vi "Autonomous Independent.vi"   [LabVIEW 2015]
doc: "This VI is called when autonomous begins, and will automatically be terminated when autonomous ends. You can carry out timed or sensor driven robot movement independently without needing to return to the caller."
uses:
  <vilib>/Rock Robotics/WPI/SafetyOutput/WPI_SafetyOutputConfigMenu.ctl
  <vilib>/Rock Robotics/Network Tables/NT Read String.vi
  <vilib>/Rock Robotics/WPI/Utilities/WPI_GetSetVariantRefNum.vi
  <vilib>/addons/control/pid/pid.llb/PID (DBL).vi
  Z navX/navX Library v2/navX Library v2.lvlib
  <vilib>/addons/control/pid/NI_PID_pid.lvlib
panel:
  # "Be sure to right-click and choose Data Operations>>Make Current Value default if you want to save the array values with the VI"
types:
  T1 = cluster{"proportional gain (Kc)":dbl, "integral time (Ti, min)":dbl, "derivative time (Td, min)":dbl}
  T2 = typedef "WPI_SafetyOutputConfigMenu.ctl" = enum16{"Enable", "Disable"}
  T3 = typedef "navX Library v2.lvlib/Z900_navX_DeviceTypeDef.ctl" = cluster{"Interface":cluster{"Protocol":T4, "Update Rate (4Hz-60Hz)":u8, "navX Open TypeDef":variant}, "Notify Packet":refnum<notifier>, "Loop VI Refnum":refnum<vi>, "Ready to Close Occurrence Refnum":refnum<k4>}
  T4 = typedef "navX Library v2.lvlib/Z900_navX_ProtocolTypeDef.ctl" = enum16{"SERIAL", "I2C", "SPI"}
  T5 = cluster{"LinearAcceleration X":dbl, "LinearAcceleration Y":dbl, "LinearAcceleration Z":dbl}
  T6 = cluster{"Velocity X":dbl, "Velocity Y":dbl, "Velocity Z":dbl, "Displacement X":dbl, "Displacement Y":dbl, "Displacement Z":dbl}
  T7 = cluster{"Yaw":dbl, "Roll":dbl, "Pitch":dbl, "Heading":dbl, "Fused Heading":dbl}
  T8 = typedef "WPI_RobotDriveDevRef.ctl" = cluster{"DevStatus":errorcluster, "Motors[]":T9[], "Square Inputs":bool, "Max Output":dbl}
  T9 = typedef "WPI_MotorControlDeviceRef.ctl" = cluster{"DeviceStatus":errorcluster, "Type":T10, "PWM":cluster{"PWM Channel":T11, "DeadBand":T12}, "CAN":cluster{"Device Number":u8, "Control Mode":T13, "Semaphore":T14, "Max Vout":dbl, "TalonSRX Control Mode":T15}, "Invert":bool}
  T10 = typedef "WPI_MotorControlType.ctl" = enum16{"PWM", "CAN", "CANTalonSRX"}
  T11 = typedef "FPGA_DIOPWMChannel.ctl" = enum8{"PWM 0", "PWM 1", "PWM 2", "PWM 3", "PWM 4", "PWM 5", "PWM 6", "PWM 7", "PWM 8", "PWM 9", "PWM MXP 0", "PWM MXP 1", "PWM MXP 2", "PWM MXP 3", "PWM MXP 4", "PWM MXP 5", "PWM MXP 6", "PWM MXP 7", "PWM MXP 8", "PWM MXP 9", "Invalid"}
  T12 = typedef "WPI_PWMDeadband.ctl" = cluster{"Name":string, "maxPositivePwm":i32, "minPositivePwm":i32, "centerPwm":i32, "maxNegativePwm":i32, "minNegativePwm":i32, "angularRange":u16}
  T13 = typedef "WPI_CANJaguar_ControlMode.ctl" = enum8{"Percent VBus", "Current", "Speed", "Position", "Voltage"}
  T14 = typedef "Semaphore RefNum" = refnum<k1>
  T15 = typedef "WPI_CANTalonSRX_APIControlMode.ctl" = enum8{"Percent VBus", "Speed", "Position", "Slave", "Unchanged / Invalid", "Voltage Compensation", "Current", "Motion Profile"}
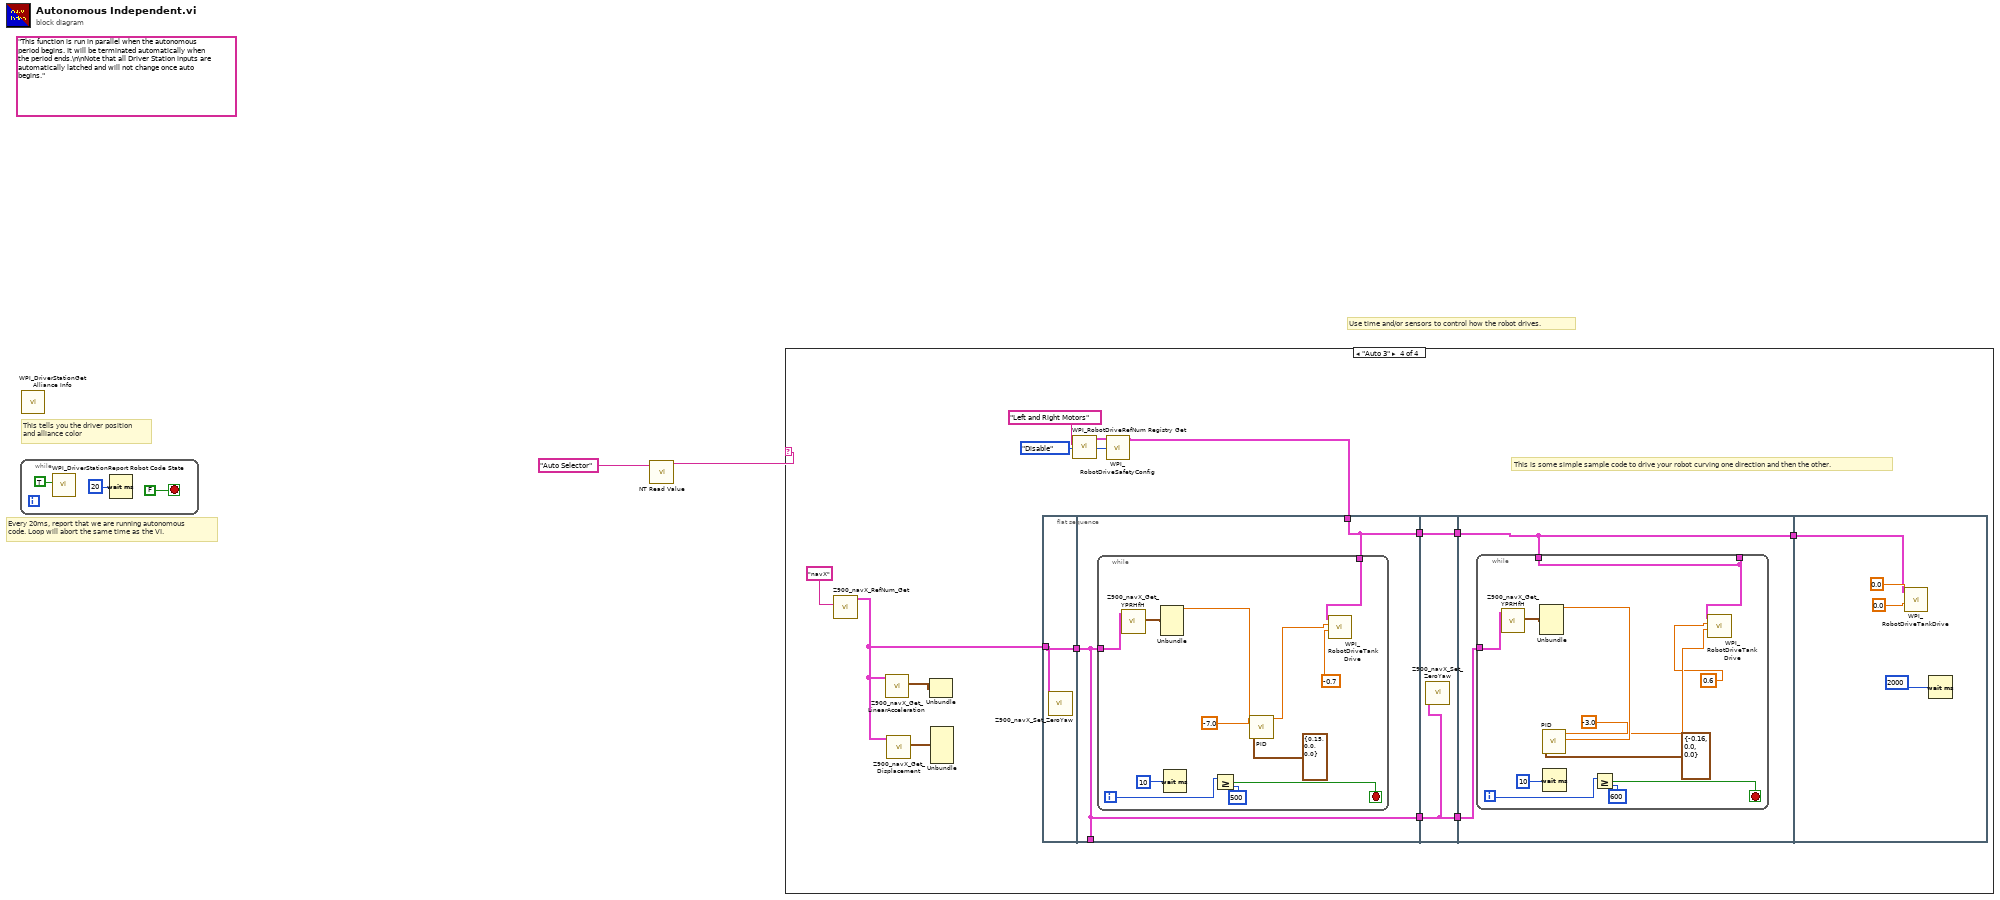
[diagram p0: block diagram]
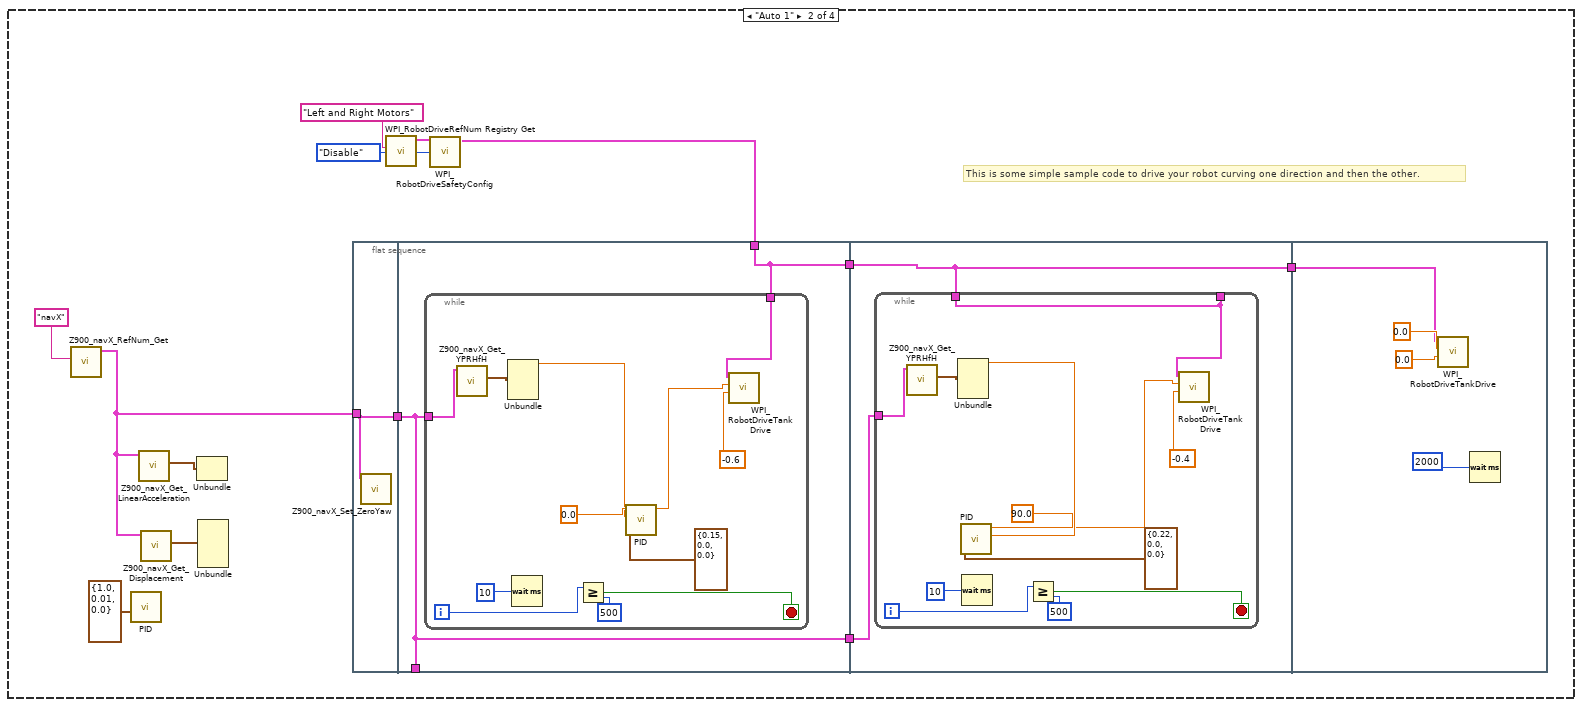
[diagram p3: hidden frame]
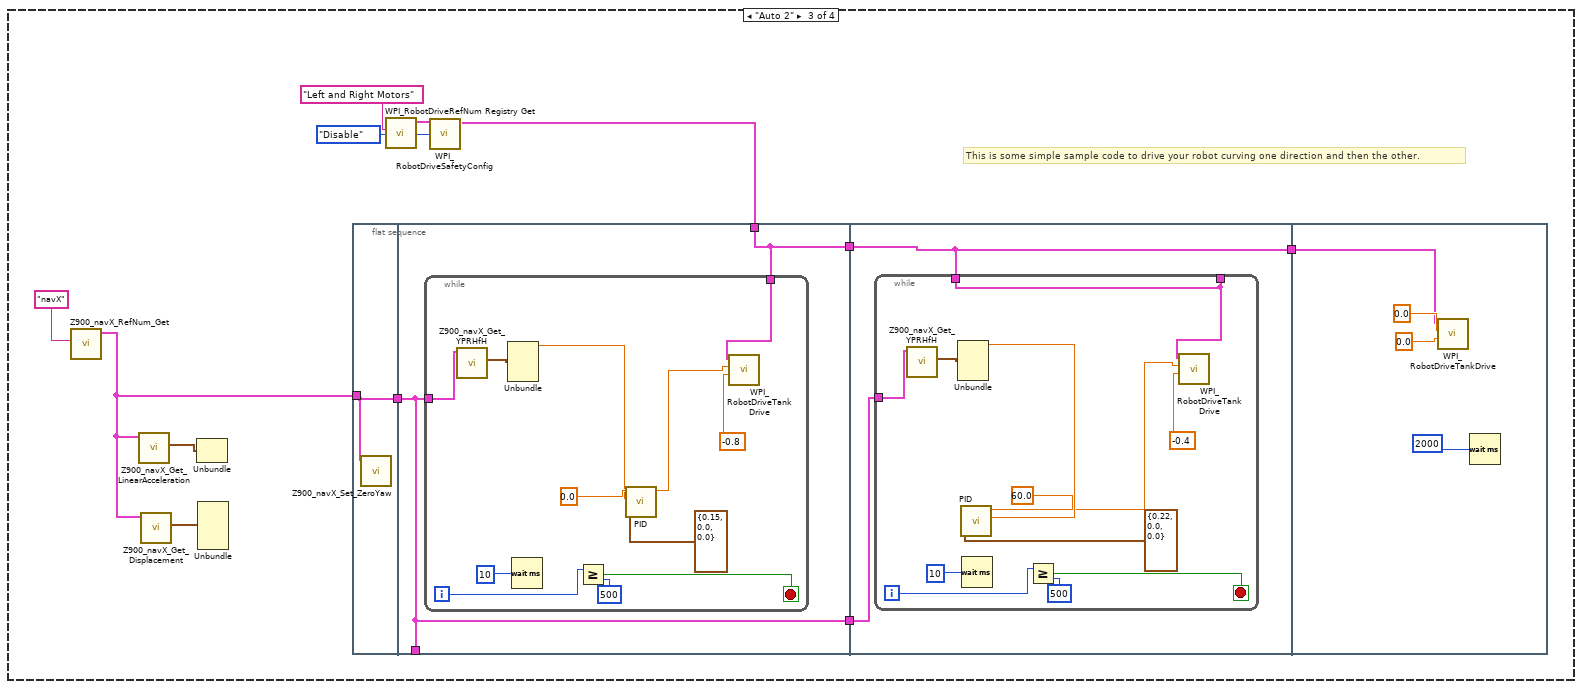
[diagram p4: hidden frame]
diagram:
  (unwired) "This function is run in parallel when the autonomous period begins. It will be terminated automatically when the period ends.\n\nNote that all Driver Station inputs are automatically latched and will not change once auto begins."
  # "Use time and/or sensors to control how the robot drives."
  # "Every 20ms, report that we are running autonomous\ncode. Loop will abort the same time as the VI."
  # "This tells you the driver position\nand alliance color"
  n1 = while {
    stop <- FALSE stop-if-true
    n2 = call <vilib>:"WPI_DriverStationReport Robot Code State.vi"("Autonomous"=TRUE) -> ()  [unwired: 10 in, 1 out]
    n3 = Wait (ms)(milliseconds to wait=u32 20) -> ()  [unwired: 1 out]
  }
  n4 = call <vilib>:"WPI_DriverStationGet Alliance Info.vi"() -> ()  [unwired: 12 out]
  n5 = call-poly <vilib>:"NT Read Value.vi"("Name"="Auto Selector") -> ("String"=w1:string)  [unwired: 9 in, 1 out]
  n6 = case shown="\"Auto 3\"" w1 {
    frame Default {
      # "You can put your main auto here, or you can right-click on the case and make any\nother frame be the default case."
      # "This is the frame that will execute if no selection is made, or if it is not recognized"
    }
    frame "Auto 1" {
      # "This is some simple sample code to drive your robot curving one direction and then the other."
      n7 = call "Z900_navX_RefNum_Get.vi"("refnum name"="navX") -> ("navX Device"=w9:T3)  [unwired: 9 in, 1 out]
      n8 = call-poly <vilib>:"PID.vi"("PID gains"=T1 {"proportional gain (Kc)"=1.0, "integral time (Ti, min)"=0.01, "derivative time (Td, min)"=0.0}) -> ()  [unwired: 9 in, 2 out]
      n9 = call "Z900_navX_Get_LinearAcceleration.vi"("navX Device"=w9) -> ("Linear Acceleration"=w11:T5)  [unwired: 7 in, 3 out]
      n10 = call "Z900_navX_Get_Displacement.vi"("navX Device"=w9) -> ("Displacement"=w10:T6)  [unwired: 7 in, 3 out]
      n11 = Unbundle(w11) -> ()  [unwired: 3 out]
      n12 = Unbundle(w10) -> ()  [unwired: 6 out]
      n13 = flat-sequence {
        tunnel: w9 -> [w19]
        tunnel: [w19] -> w7
        tunnel: w14 -> [w21]
        tunnel: [w21] -> w18
        tunnel: w7 -> [w20]
        tunnel: [w20] -> _
        tunnel: [w20] -> w6
        tunnel: w18 -> [w35]
        tunnel: [w35] -> w13
        tunnel: w6 -> [w34]
        tunnel: w13 -> [w48]
        frame #0 {
          n14 = call "Z900_navX_Set_ZeroYaw.vi"("navX Device"=w19) -> ()  [unwired: 9 in, 2 out]
        }
        frame #1 {
          n15 = while {
            tunnel: w21 -> [w30]
            tunnel: w20 -> [w25]
            i -> [w29]
            stop <- w27 stop-if-true
            n16 = call "Z900_navX_Get_YPRHfH.vi"("navX Device"=w25) -> ("YRPHfH"=w26:T7)  [unwired: 7 in, 3 out]
            n17 = Unbundle(w26) -> ("Yaw"=w22:dbl)  [unwired: 4 out]
            n18 = Wait (ms)(milliseconds to wait=10) -> ()  [unwired: 1 out]
            n19 = Greater Or Equal?(x=w29, y=500) -> (x >= y?=w27:bool)
            n20 = call-poly <vilib>:"PID.vi"("PID gains"=T1 {"proportional gain (Kc)"=0.15, "integral time (Ti, min)"=0.0, "derivative time (Td, min)"=0.0}, "process variable"=w22, "setpoint"=0.0) -> ("output"=w23:dbl)  [unwired: 7 in, 1 out]
            n21 = call <vilib>:"WPI_RobotDriveTankDrive.vi"("Right axis value"=-0.6, "Left axis value"=w23, "RobotDriveDevRef"=w30) -> ()  [unwired: 6 in, 3 out]
          }
        }
        frame #2 {
          n22 = while {
            tunnel: [w36] -> _
            tunnel: w34 -> [w39]
            tunnel: w35 -> [w36]
            i -> [w44]
            stop <- w42 stop-if-true
            n23 = call "Z900_navX_Get_YPRHfH.vi"("navX Device"=w39) -> ("YRPHfH"=w41:T7)  [unwired: 7 in, 3 out]
            n24 = Unbundle(w41) -> ("Yaw"=w40:dbl)  [unwired: 4 out]
            n25 = call-poly <vilib>:"PID.vi"("PID gains"=T1 {"proportional gain (Kc)"=0.22, "integral time (Ti, min)"=0.0, "derivative time (Td, min)"=0.0}, "process variable"=w40, "setpoint"=90.0) -> ("output"=w37:dbl)  [unwired: 7 in, 1 out]
            n26 = Wait (ms)(milliseconds to wait=10) -> ()  [unwired: 1 out]
            n27 = Greater Or Equal?(x=w44, y=500) -> (x >= y?=w42:bool)
            n28 = call <vilib>:"WPI_RobotDriveTankDrive.vi"("Right axis value"=-0.4, "Left axis value"=w37, "RobotDriveDevRef"=w36) -> ()  [unwired: 6 in, 3 out]
          }
        }
        frame #3 {
          n29 = call <vilib>:"WPI_RobotDriveTankDrive.vi"("Right axis value"=0.0, "Left axis value"=0.0, "RobotDriveDevRef"=w48) -> ()  [unwired: 6 in, 3 out]
          n30 = Wait (ms)(milliseconds to wait=2000) -> ()  [unwired: 1 out]
        }
      }
      n31 = call <vilib>:"WPI_RobotDriveRefNum Registry Get.vi"("refnum name"="Left and Right Motors") -> ("RobotDriveDevRef"=w15:T8)  [unwired: 9 in, 1 out]
      n32 = call <vilib>:"WPI_RobotDriveSafetyConfig.vi"("mode"=WPI_SafetyOutputConfigMenu."Disable", "RobotDriveDevRef"=w15) -> ("RobotDriveDevRef"=w14:T8)  [unwired: 8 in, 1 out]
    }
    frame "Auto 2" {
      # "This is some simple sample code to drive your robot curving one direction and then the other."
      n33 = call "Z900_navX_RefNum_Get.vi"("refnum name"="navX") -> ("navX Device"=w52:T3)  [unwired: 9 in, 1 out]
      n34 = call "Z900_navX_Get_LinearAcceleration.vi"("navX Device"=w52) -> ("Linear Acceleration"=w54:T5)  [unwired: 7 in, 3 out]
      n35 = call "Z900_navX_Get_Displacement.vi"("navX Device"=w52) -> ("Displacement"=w53:T6)  [unwired: 7 in, 3 out]
      n36 = Unbundle(w54) -> ()  [unwired: 3 out]
      n37 = Unbundle(w53) -> ()  [unwired: 6 out]
      n38 = flat-sequence {
        tunnel: w52 -> [w64]
        tunnel: [w64] -> w63
        tunnel: w56 -> [w66]
        tunnel: [w66] -> w62
        tunnel: w63 -> [w65]
        tunnel: [w65] -> _
        tunnel: [w65] -> w61
        tunnel: w62 -> [w80]
        tunnel: [w80] -> w60
        tunnel: w61 -> [w79]
        tunnel: w60 -> [w93]
        frame #0 {
          n39 = call "Z900_navX_Set_ZeroYaw.vi"("navX Device"=w64) -> ()  [unwired: 9 in, 2 out]
        }
        frame #1 {
          n40 = while {
            tunnel: w66 -> [w75]
            tunnel: w65 -> [w70]
            i -> [w74]
            stop <- w72 stop-if-true
            n41 = call "Z900_navX_Get_YPRHfH.vi"("navX Device"=w70) -> ("YRPHfH"=w71:T7)  [unwired: 7 in, 3 out]
            n42 = Unbundle(w71) -> ("Yaw"=w67:dbl)  [unwired: 4 out]
            n43 = Wait (ms)(milliseconds to wait=10) -> ()  [unwired: 1 out]
            n44 = Greater Or Equal?(x=w74, y=500) -> (x >= y?=w72:bool)
            n45 = call-poly <vilib>:"PID.vi"("PID gains"=T1 {"proportional gain (Kc)"=0.15, "integral time (Ti, min)"=0.0, "derivative time (Td, min)"=0.0}, "process variable"=w67, "setpoint"=0.0) -> ("output"=w68:dbl)  [unwired: 7 in, 1 out]
            n46 = call <vilib>:"WPI_RobotDriveTankDrive.vi"("Right axis value"=-0.8, "Left axis value"=w68, "RobotDriveDevRef"=w75) -> ()  [unwired: 6 in, 3 out]
          }
        }
        frame #2 {
          n47 = while {
            tunnel: [w81] -> _
            tunnel: w79 -> [w84]
            tunnel: w80 -> [w81]
            i -> [w89]
            stop <- w87 stop-if-true
            n48 = call "Z900_navX_Get_YPRHfH.vi"("navX Device"=w84) -> ("YRPHfH"=w86:T7)  [unwired: 7 in, 3 out]
            n49 = Unbundle(w86) -> ("Yaw"=w85:dbl)  [unwired: 4 out]
            n50 = call-poly <vilib>:"PID.vi"("PID gains"=T1 {"proportional gain (Kc)"=0.22, "integral time (Ti, min)"=0.0, "derivative time (Td, min)"=0.0}, "process variable"=w85, "setpoint"=60.0) -> ("output"=w82:dbl)  [unwired: 7 in, 1 out]
            n51 = Wait (ms)(milliseconds to wait=10) -> ()  [unwired: 1 out]
            n52 = Greater Or Equal?(x=w89, y=500) -> (x >= y?=w87:bool)
            n53 = call <vilib>:"WPI_RobotDriveTankDrive.vi"("Right axis value"=-0.4, "Left axis value"=w82, "RobotDriveDevRef"=w81) -> ()  [unwired: 6 in, 3 out]
          }
        }
        frame #3 {
          n54 = call <vilib>:"WPI_RobotDriveTankDrive.vi"("Right axis value"=0.0, "Left axis value"=0.0, "RobotDriveDevRef"=w93) -> ()  [unwired: 6 in, 3 out]
          n55 = Wait (ms)(milliseconds to wait=2000) -> ()  [unwired: 1 out]
        }
      }
      n56 = call <vilib>:"WPI_RobotDriveRefNum Registry Get.vi"("refnum name"="Left and Right Motors") -> ("RobotDriveDevRef"=w57:T8)  [unwired: 9 in, 1 out]
      n57 = call <vilib>:"WPI_RobotDriveSafetyConfig.vi"("mode"=WPI_SafetyOutputConfigMenu."Disable", "RobotDriveDevRef"=w57) -> ("RobotDriveDevRef"=w56:T8)  [unwired: 8 in, 1 out]
    }
    frame "Auto 3" {
      # "This is some simple sample code to drive your robot curving one direction and then the other."
      n58 = call "Z900_navX_RefNum_Get.vi"("refnum name"="navX") -> ("navX Device"=w101:T3)  [unwired: 9 in, 1 out]
      n59 = call "Z900_navX_Get_LinearAcceleration.vi"("navX Device"=w101) -> ("Linear Acceleration"=w103:T5)  [unwired: 7 in, 3 out]
      n60 = call "Z900_navX_Get_Displacement.vi"("navX Device"=w101) -> ("Displacement"=w102:T6)  [unwired: 7 in, 3 out]
      n61 = Unbundle(w103) -> ()  [unwired: 3 out]
      n62 = Unbundle(w102) -> ()  [unwired: 6 out]
      n63 = flat-sequence {
        tunnel: w101 -> [w111]
        tunnel: [w111] -> w110
        tunnel: w105 -> [w113]
        tunnel: [w113] -> w100
        tunnel: w110 -> [w112]
        tunnel: [w112] -> _
        tunnel: [w112] -> w98
        tunnel: w100 -> [w127]
        tunnel: [w127] -> w99
        tunnel: w98 -> [w126]
        tunnel: [w126] -> w97
        tunnel: w99 -> [w129]
        tunnel: [w129] -> w109
        tunnel: w97 -> [w128]
        tunnel: w109 -> [w142]
        frame #0 {
          n64 = call "Z900_navX_Set_ZeroYaw.vi"("navX Device"=w111) -> ()  [unwired: 9 in, 2 out]
        }
        frame #1 {
          n65 = while {
            tunnel: w113 -> [w122]
            tunnel: w112 -> [w117]
            i -> [w121]
            stop <- w119 stop-if-true
            n66 = call "Z900_navX_Get_YPRHfH.vi"("navX Device"=w117) -> ("YRPHfH"=w118:T7)  [unwired: 7 in, 3 out]
            n67 = Unbundle(w118) -> ("Yaw"=w114:dbl)  [unwired: 4 out]
            n68 = Wait (ms)(milliseconds to wait=10) -> ()  [unwired: 1 out]
            n69 = Greater Or Equal?(x=w121, y=500) -> (x >= y?=w119:bool)
            n70 = call-poly <vilib>:"PID.vi"("PID gains"=T1 {"proportional gain (Kc)"=0.15, "integral time (Ti, min)"=0.0, "derivative time (Td, min)"=0.0}, "process variable"=w114, "setpoint"=-7.0) -> ("output"=w115:dbl)  [unwired: 7 in, 1 out]
            n71 = call <vilib>:"WPI_RobotDriveTankDrive.vi"("Right axis value"=-0.7, "Left axis value"=w115, "RobotDriveDevRef"=w122) -> ()  [unwired: 6 in, 3 out]
          }
        }
        frame #2 {
          n72 = call "Z900_navX_Set_ZeroYaw.vi"("navX Device"=w126) -> ()  [unwired: 9 in, 2 out]
        }
        frame #3 {
          n73 = while {
            tunnel: [w132] -> _
            tunnel: w128 -> [w133]
            tunnel: w129 -> [w132]
            i -> [w138]
            stop <- w136 stop-if-true
            n74 = call "Z900_navX_Get_YPRHfH.vi"("navX Device"=w133) -> ("YRPHfH"=w135:T7)  [unwired: 7 in, 3 out]
            n75 = Unbundle(w135) -> ("Yaw"=w134:dbl)  [unwired: 4 out]
            n76 = call-poly <vilib>:"PID.vi"("PID gains"=T1 {"proportional gain (Kc)"=-0.16, "integral time (Ti, min)"=0.0, "derivative time (Td, min)"=0.0}, "process variable"=w134, "setpoint"=-3.0) -> ("output"=w131:dbl)  [unwired: 7 in, 1 out]
            n77 = Wait (ms)(milliseconds to wait=10) -> ()  [unwired: 1 out]
            n78 = Greater Or Equal?(x=w138, y=600) -> (x >= y?=w136:bool)
            n79 = call <vilib>:"WPI_RobotDriveTankDrive.vi"("Right axis value"=w131, "Left axis value"=0.6, "RobotDriveDevRef"=w132) -> ()  [unwired: 6 in, 3 out]
          }
        }
        frame #4 {
          n80 = call <vilib>:"WPI_RobotDriveTankDrive.vi"("Right axis value"=0.0, "Left axis value"=0.0, "RobotDriveDevRef"=w142) -> ()  [unwired: 6 in, 3 out]
          n81 = Wait (ms)(milliseconds to wait=2000) -> ()  [unwired: 1 out]
        }
      }
      n82 = call <vilib>:"WPI_RobotDriveRefNum Registry Get.vi"("refnum name"="Left and Right Motors") -> ("RobotDriveDevRef"=w106:T8)  [unwired: 9 in, 1 out]
      n83 = call <vilib>:"WPI_RobotDriveSafetyConfig.vi"("mode"=WPI_SafetyOutputConfigMenu."Disable", "RobotDriveDevRef"=w106) -> ("RobotDriveDevRef"=w105:T8)  [unwired: 8 in, 1 out]
    }
  }
